vi "RH_PPMU_Set0V.vi"(8 "error in":errorcluster, 9 "Settling (ms)":u32, 10 "channel list":string, 11 "PPMU Session In":refnum<k15>) -> (0 "error out":errorcluster, 3 "PPMU Session Out":refnum<k15>)   [LabVIEW 2023, in "ResourceHandling.lvlib"]
doc: "Set 0V, start sourcing and waits a settling times"
uses:
  ResourceHandling.lvlib
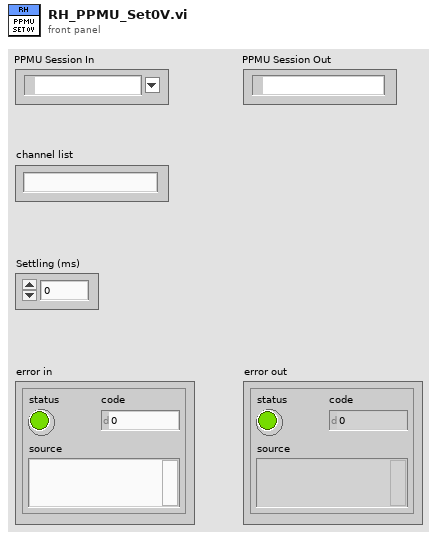
[diagram p1: front panel]
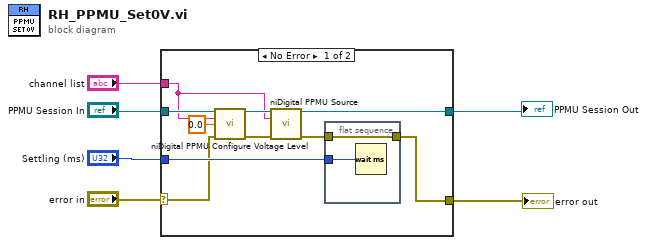
[diagram p0: block diagram]
diagram:
  n1 = case shown="No Error" "error in" {
    selector: "error in" -> [w7 w20]
    tunnel: "PPMU Session In" -> [w16 w19]
    tunnel: "channel list" -> [w12 _]
    tunnel: [w10 w20] -> w3
    tunnel: [w9 w19] -> w2
    tunnel: "Settling (ms)" -> [w8 _]
    frame No Error {
      n2 = call <instrlib>:"niDigital PPMU Configure Voltage Level.vi"("instrument handle"=w16, "channel list"=w12, "voltage level (V)"=0.0, "error in"=w7) -> ("instrument handle out"=w14:refnum<k15>, "error out"=w13:errorcluster)  [unwired: 10 in]
      n3 = call <instrlib>:"niDigital PPMU Source.vi"("instrument handle"=w14, "channel list"=w12, "error in"=w13) -> ("instrument handle out"=w9:refnum<k15>, "error out"=w11:errorcluster)  [unwired: 11 in]
      n4 = flat-sequence {
        tunnel: w11 -> [w18]
        tunnel: [w18] -> w10
        tunnel: w8 -> [w17]
        frame #0 {
          n5 = Wait (ms)(milliseconds to wait=w17) -> ()  [unwired: 1 out]
        }
      }
    }
    frame Error {
    }
  }
  "PPMU Session Out" <- w2
  "error out" <- w3
